vi "TreatFiles.vi"(7 "Directory(T)":bool=TRUE, 8 "error in (no error)":errorcluster, 11 "Top Level Directory":path) -> (0 "error out":errorcluster)   [LabVIEW 2014]
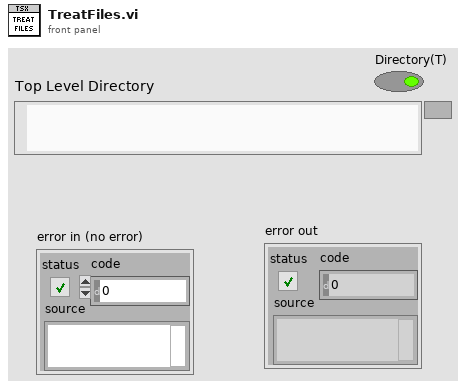
[diagram p1: front panel]
types:
  T1 = enum32{"invalid lock state", "Not Locked", "Locked (No Password)", "Password-protected"}
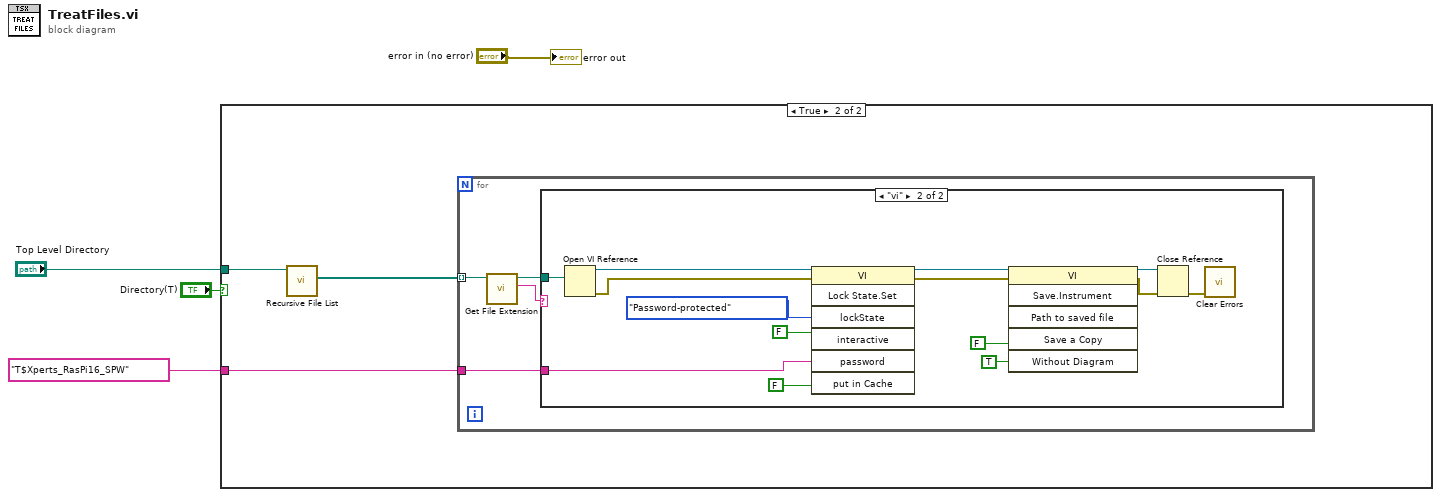
[diagram p0: block diagram]
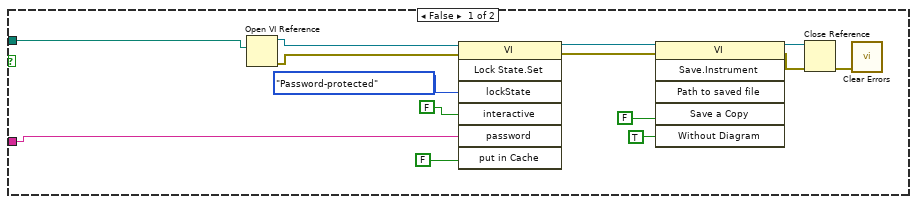
[diagram p2: hidden frame]
diagram:
  n1 = case shown="True" "Directory(T)" {
    tunnel: "Top Level Directory" -> [w6 w21]
    tunnel: "T$Xperts_RasPi16_SPW" ("Password") -> [w5 w19]
    frame False {
      n2 = Open VI Reference(vi path=w6) -> (vi reference=w17:refnum<vi>, error out=w18:errorcluster)  [unwired: 5 in]
      n3 = invoke class="VI" method="Lock State.Set"(reference=w17, error in=w18, "lockState"=T1."Password-protected" ("Lock State"), "interactive"=FALSE ("Interactive"), "password"=w5, "put in Cache"=FALSE ("Put in Cache")) -> (reference out=w10:refnum<vi>, error out=w11:errorcluster)  [unwired: 1 in, 5 out]
      n4 = invoke class="VI" method="Save.Instrument"(reference=w10, error in=w11, "Save a Copy"=FALSE, "Without Diagram"=TRUE) -> (reference out=w15:refnum<vi>, error out=w16:errorcluster)  [unwired: 2 in, 4 out]
      n5 = Close Reference(reference=w15, error in (no error)=w16) -> (error out=w14:errorcluster)
      n6 = call <vilib>:"Clear Errors.vi"("error in (no error)"=w14) -> ()  [unwired: 5 in, 2 out]
    }
    frame True {
      n7 = call <vilib>:"Recursive File List.vi"("Folder Path"=w21) -> ("All Files in Dir"=w20:path[])  [unwired: 6 in, 4 out]
      n8 = for {
        tunnel: w20 -> [w25] mode=indexing
        tunnel: w19 -> [w22]
        n9 = call <vilib>:"Get File Extension.vi"("file"=w25) -> ("lowercase file extension"=w24:string, "dup file"=w23:path)  [unwired: 7 in, 2 out]
        n10 = case shown="\"vi\"" w24 {
          tunnel: w23 -> [_ w34]
          tunnel: w22 -> [_ w35]
          frame "False", Default {
          }
          frame "vi" {
            n11 = Open VI Reference(vi path=w34) -> (vi reference=w36:refnum<vi>, error out=w39:errorcluster)  [unwired: 5 in]
            n12 = invoke class="VI" method="Lock State.Set"(reference=w36, error in=w39, "lockState"=T1."Password-protected" ("Lock State"), "interactive"=FALSE ("Interactive"), "password"=w35, "put in Cache"=FALSE ("Put in Cache")) -> (reference out=w29:refnum<vi>, error out=w30:errorcluster)  [unwired: 1 in, 5 out]
            n13 = invoke class="VI" method="Save.Instrument"(reference=w29, error in=w30, "Save a Copy"=FALSE, "Without Diagram"=TRUE) -> (reference out=w37:refnum<vi>, error out=w38:errorcluster)  [unwired: 2 in, 4 out]
            n14 = Close Reference(reference=w37, error in (no error)=w38) -> (error out=w33:errorcluster)
            n15 = call <vilib>:"Clear Errors.vi"("error in (no error)"=w33) -> ()  [unwired: 5 in, 2 out]
          }
        }
      }
    }
  }
  "error out" <- "error in (no error)"
